vi "SubTemplate_4x4x4_New.vi"(6 "User counter":bool, 7 "Create method":T1(ring), 8 "error in (no error)":errorcluster, 10 "Object name":string, 11 "reference in":refnum<class "SubTemplate_4x4x4.lvclass">) -> (0 "error out":errorcluster, 1 "First user":bool, 2 "# of objects":i32, 3 "reference out":refnum<class "SubTemplate_4x4x4.lvclass">)   [LabVIEW 2020, in "SubTemplate_4x4x4.lvclass"]
doc: "Looks up an existing object matching object name or creates a new object and returns a refnum you can use when calling other class methods.\n\nObjects created with this VI should be destroyed using this class Delete VI."
uses:
  SubTemplate_4x4x4.lvclass
  vi.lib/addons/_goop3.llb/3GOOPStates.ctl
  SubTemplate_4x4x4.lvclass/SubTemplate_4x4x4.ctl
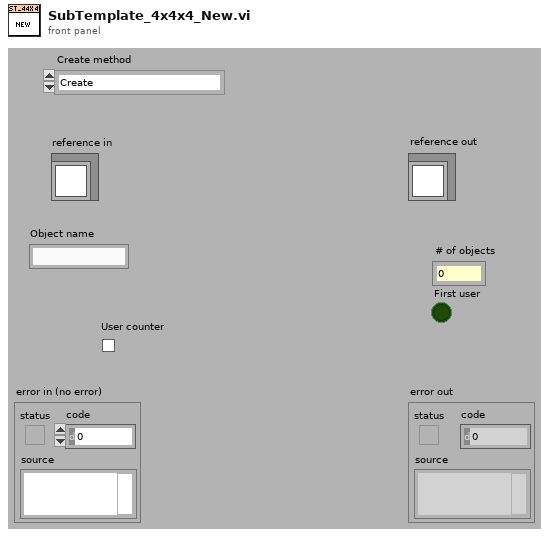
[diagram p1: front panel]
types:
  T1 = enum16{"Create", "Create or look up existing", "Look up existing"}
  T2 = typedef "3GOOPStates.ctl" = enum16{"Set", "Get", "New", "Delete", "Clear", "Test and get", "Unlock data", "Information", "Look up existing", "New or look up existing", "Test and get shared", "Get shared", "Set shared", "Unlock shared", "Find dynamic method", "Register dynamic method", "Preload dynamic method", "Probe", "Cast to more generic", "Cast to more specific"}
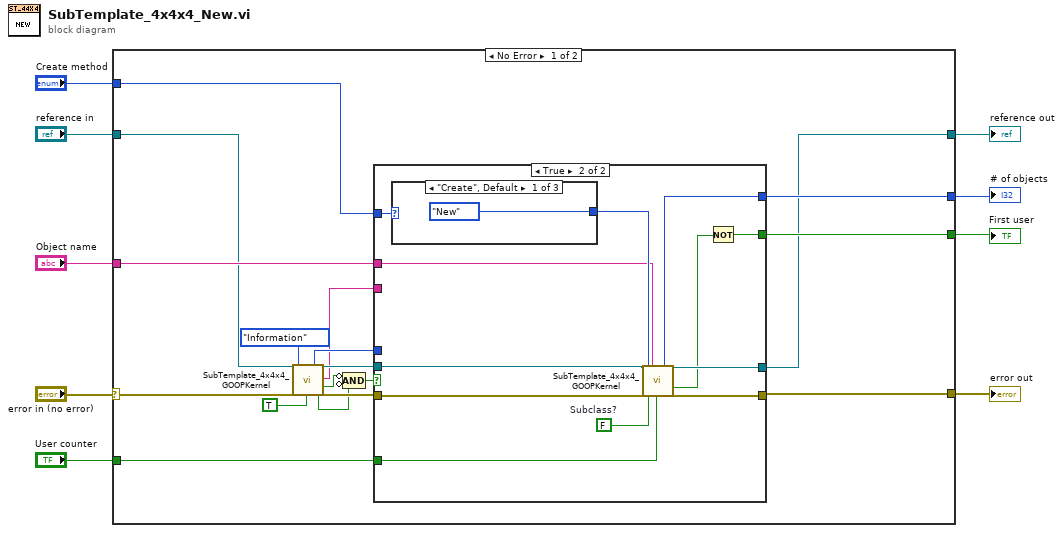
[diagram p0: block diagram]
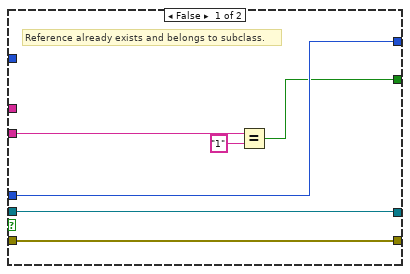
[diagram p2: hidden frame]
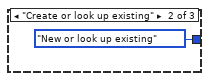
[diagram p3: hidden frame]
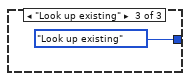
[diagram p4: hidden frame]
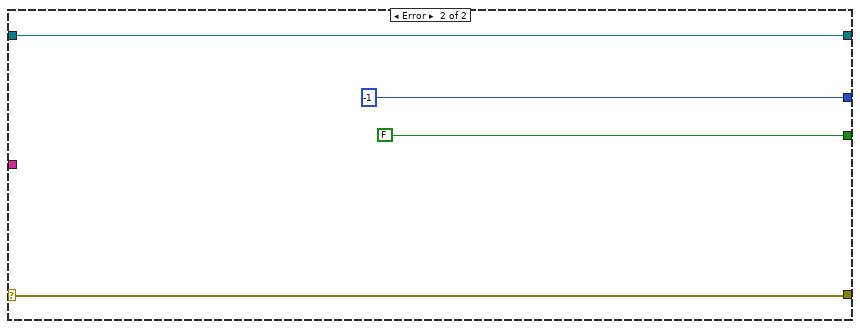
[diagram p5: hidden frame]
diagram:
  n1 = case shown="No Error" "error in (no error)" {
    selector: "error in (no error)" -> [w17 w51]
    tunnel: [w13 w51] -> w9
    tunnel: [w26 -1 ("Nr of open handles")] -> w8
    tunnel: "Object name" -> [w25 _]
    tunnel: "Create method" -> [w27 _]
    tunnel: "reference in" -> [w12 w50]
    tunnel: [w11 w50] -> w3
    tunnel: [w16 FALSE] -> w2
    tunnel: "User counter" -> [w15 _]
    frame No Error {
      n2 = call "SubTemplate_4x4x4_GOOPKernel.vi"("Ref in"=w12, "error in (no error)"=w17, "Action"=3GOOPStates."Information", "Misc"=TRUE) -> ("# of objects"=w20:i32, "IsSubclass?"=w23:bool, "Ref out"=w18:refnum<class "SubTemplate_4x4x4.lvclass">, "Probe out"=w14:string, "Exists?"=w22:bool, "error out"=w24:errorcluster)  [unwired: 13 in, 5 out]
      n3 = Compound Arithmetic op=AND(invert w22, invert w23) -> (w21:bool)
      n4 = case shown="True" w21 {
        tunnel: w27 -> [_ w45]
        tunnel: [w31 w37] -> w11
        tunnel: w24 -> [w33 w39]
        tunnel: [w33 w44] -> w13
        tunnel: [w32 w40] -> w26
        tunnel: w25 -> [_ w41]
        tunnel: w20 -> [w32 _]
        tunnel: w18 -> [w31 w38]
        tunnel: [w28 w35] -> w16
        tunnel: w15 -> [_ w34]
        tunnel: w14 -> [w30 _]
        frame False {
          # "Reference already exists and belongs to subclass."
          n5 = Equal?(x=w30, y="1") -> (x = y?=w28:bool)
        }
        frame True {
          w42 = FALSE  # Subclass?
          n6 = case shown="\"Create\", Default" w45 {
            tunnel: [3GOOPStates."New" ("Action") 3GOOPStates."New or look up existing" ("Action") 3GOOPStates."Look up existing" ("Action")] -> w43
            frame "Create", Default {
            }
            frame "Create or look up existing" {
            }
            frame "Look up existing" {
            }
          }
          n7 = call "SubTemplate_4x4x4_GOOPKernel.vi"("Ref in"=w38, "error in (no error)"=w39, "Action"=w43, "Subclass?"=w42, "Object name"=w41, "Misc"=w34) -> ("# of objects"=w40:i32, "Ref out"=w37:refnum<class "SubTemplate_4x4x4.lvclass">, "Exists?"=w36:bool, "error out"=w44:errorcluster)  [unwired: 11 in, 7 out]
          n8 = Not(x=w36) -> (.not. x?=w35:bool)
        }
      }
    }
    frame Error {
    }
  }
  "error out" <- w9
  "# of objects" <- w8
  "reference out" <- w3
  "First user" <- w2
